vi "test_DigitalInstrument_InitializeSessionsWithUnregisteredSessionsReserved_RemoteSessionsInitialized.vi"(8 "error in":errorcluster) -> (0 "error out":errorcluster, 2 "result":string, 3 "pass":bool)   [LabVIEW 2020, in "MeasurementServerTests.lvlib"]
uses:
  MeasurementServerTests.lvlib
  78c0f8c1-8fe2-4936-9d85-28ac64cefb56.vi
  Runtime/MeasurementLink niDigital/Initialize Sessions - NSess.vi
  Runtime/MeasurementLink niDigital/MeasurementLink niDigital.lvlib
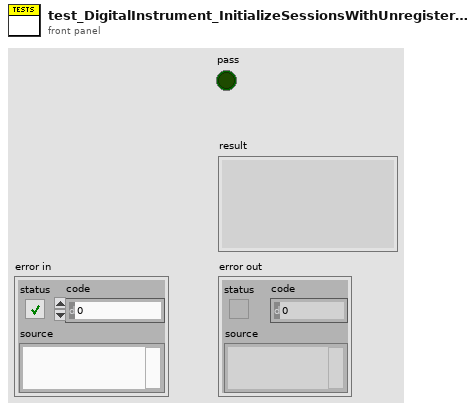
[diagram p1: front panel]
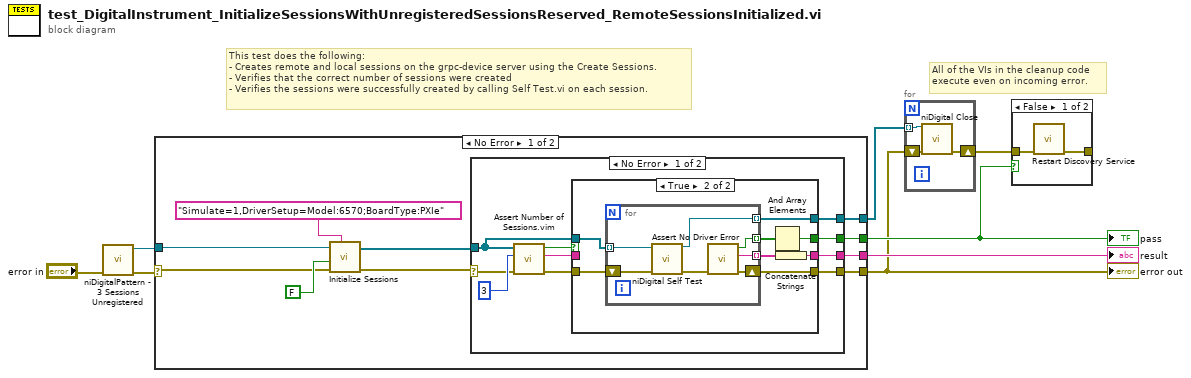
[diagram p0: block diagram]
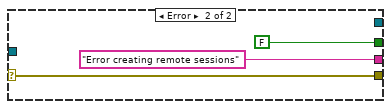
[diagram p3: hidden frame]
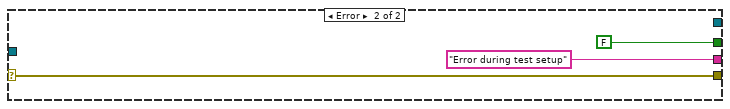
[diagram p4: hidden frame]
diagram:
  # "All of the VIs in the cleanup code\nexecute even on incoming error."
  # "This test does the following:\n- Creates remote and local sessions on the grpc-device server using the Create Sessions.\n- Verifies that the correct number of sessions were created\n- Verifies the sessions were successfully created by calling Self Test.vi on each session."
  n1 = call "niDigitalPattern - 3 Sessions Unregistered.vi"("error in (no error)"="error in") -> ("error out"=w3:errorcluster, "Session Reservation out"=w2:refnum<class "Session Reservation.lvclass">)  [unwired: 9 in]
  n2 = case shown="No Error" w3 {
    selector: w3 -> [w13 w51]
    tunnel: [w17 w51] -> w4
    tunnel: [w18 FALSE] -> w5
    tunnel: [w16 "Error during test setup" ("f")] -> w8
    tunnel: [w15 _] -> w7
    tunnel: w2 -> [w12 _]
    frame No Error {
      n3 = call-poly "Initialize Sessions.vi"("option string"="Simulate=1,DriverSetup=Model:6570;BoardType:PXIe", "error in"=w13, "reset"=FALSE, "session reservation in"=w12) -> ("error out"=w10:errorcluster, "sessions"=w11:refnum<k15>[])  [unwired: 4 in, 2 out]
      n4 = case shown="No Error" w10 {
        selector: w10 -> [w23 w49]
        tunnel: [w24 FALSE] -> w18
        tunnel: [w27 w49] -> w17
        tunnel: [w28 "Error creating remote sessions"] -> w16
        tunnel: [w26 _] -> w15
        tunnel: w11 -> [w19 _]
        frame No Error {
          n5 = call "Assert Number of Sessions.vim"("error in"=w23, "expected number of sessions"=3 ("y"), "sessions"=w19) -> ("error out"=w22:errorcluster, "result"=w20:string, "pass"=w21:bool)  [unwired: 6 in]
          n6 = case shown="True" w21 {
            selector: w21 -> [w32 _]
            tunnel: [w31 w33] -> w28
            tunnel: [w30 w38] -> w27
            tunnel: [w29 w37] -> w26
            tunnel: w19 -> [w29 w36]
            tunnel: [w32 w34] -> w24
            tunnel: w22 -> [w30 w35]
            tunnel: w20 -> [w31 _]
            frame False {
            }
            frame True {
              n7 = for {
                tunnel: [w47] -> w40 mode=indexing
                tunnel: [w46] -> w39 mode=indexing
                tunnel: [w44] -> w37 mode=indexing
                tunnel: w36 -> [w42] mode=indexing
                shift-right: [w45] -> w38
                shift-left: w35 -> [w41]
                n8 = call <instrlib>:"niDigital Self Test.vi"("instrument handle in"=w42, "error in"=w41) -> ("instrument handle out"=w44:refnum<k15>, "error out"=w43:errorcluster)  [unwired: 10 in, 2 out]
                n9 = call "Assert No Driver Error.vi"("error in"=w43) -> ("error out"=w45:errorcluster, "result"=w46:string, "pass?"=w47:bool)  [unwired: 8 in]
              }
              n10 = And Array Elements(Boolean array=w40) -> (logical AND=w34:bool)
              n11 = Concatenate Strings(w39) -> (w33:string)
            }
          }
        }
        frame Error {
        }
      }
    }
    frame Error {
    }
  }
  "error out" <- w4
  "pass" <- w5
  "result" <- w8
  n12 = for {
    tunnel: w7 -> [w56] mode=indexing
    shift-right: [w55] -> w6
    shift-left: w4 -> [w54]
    n13 = call <instrlib>:"niDigital Close.vi"("instrument handle"=w56, "error in"=w54) -> ("error out"=w55:errorcluster)  [unwired: 13 in]
  }
  n14 = case shown="False" w5 {
    tunnel: w6 -> [w58 _]
    tunnel: [w57 _] -> _
    frame False {
      n15 = call "Restart Discovery Service.vi"("error in"=w58) -> ("error out"=w57:errorcluster)  [unwired: 10 in]
    }
    frame True {
    }
  }
